vi "Sensor Send to Dash.vi"   [LabVIEW 2014]
uses:
  Global Variables/Sensor Data (Edited).vi
  <vilib>/Rock Robotics/Network Tables/SD Write Number.vi
  <vilib>/Rock Robotics/Network Tables/SD Write Boolean Array.vi
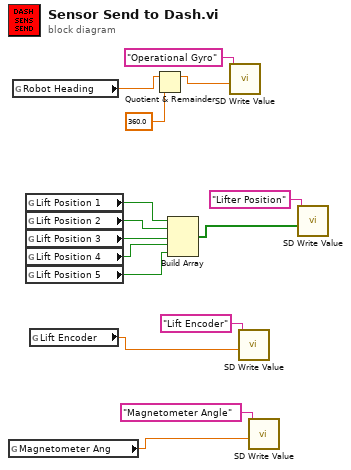
[diagram p0: block diagram]
diagram:
  n1 = global read "Sensor Data (Edited).vi" "Magnetometer Ang"() -> (w1:dbl)
  n2 = global read "Sensor Data (Edited).vi" "Robot Heading"() -> (w14:dbl)
  n3 = global read "Sensor Data (Edited).vi" "Lift Position 1"() -> (w11:bool)
  n4 = global read "Sensor Data (Edited).vi" "Lift Position 2"() -> (w10:bool)
  n5 = global read "Sensor Data (Edited).vi" "Lift Position 3"() -> (w9:bool)
  n6 = global read "Sensor Data (Edited).vi" "Lift Position 4"() -> (w7:bool)
  n7 = global read "Sensor Data (Edited).vi" "Lift Position 5"() -> (w8:bool)
  n8 = global read "Sensor Data (Edited).vi" "Lift Encoder"() -> (w3:dbl)
  n9 = Quotient & Remainder(x=w14, y=360.0 ("upper limit")) -> (x-y*floor(x/y)=w12:dbl)  [unwired: 1 out]
  n10 = Build Array(w11, w10, w9, w7, w8) -> (w6:bool[])
  n11 = call-poly <vilib>:"SD Write Value.vi"("Numeric"=w12, "Name"="Operational Gyro") -> ()  [unwired: 8 in, 2 out]
  n12 = call-poly <vilib>:"SD Write Value.vi"("Numeric"=w3, "Name"="Lift Encoder") -> ()  [unwired: 8 in, 2 out]
  n13 = call-poly <vilib>:"SD Write Value.vi"("Numeric"=w1, "Name"="Magnetometer Angle") -> ()  [unwired: 8 in, 2 out]
  n14 = call-poly <vilib>:"SD Write Value.vi"("Boolean Array"=w6, "Name"="Lifter Position") -> ()  [unwired: 8 in, 2 out]
